vi "macro_LinearSystem_Sim_Execute.vi"() -> ()   [LabVIEW 2019, in "Trajectory_Library.lvlib"]
uses:
  BatterySim_CalculateLoadedBatteryVoltage.vi
  Trajectory_Library.lvlib
  <vilib>/Analysis/Matrix/Datatypes/RealMatrix.ctl
  <vilib>/Analysis/Matrix/NI_Matrix.lvlib
  TypeDef/LINEAR_SYSTEM.ctl
panel:
  in  "Demand Array (CO)":dbl[](array[numeric])
  in  "Linear System":T1
  in  "Current":dbl
  # "<States,States>"
  # "<States,Inputs>"
  # "<Outputs,States>"
  # "<Outputs,Inputs>"
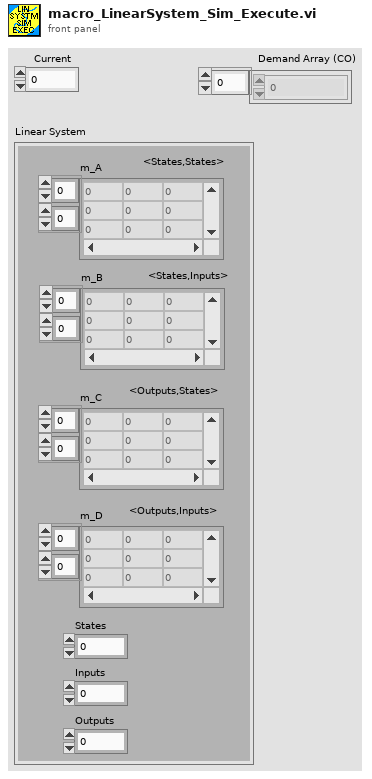
[diagram p1: front panel]
types:
  T1 = typedef "Trajectory_Library.lvlib/LINEAR_SYSTEM.ctl" = cluster{"m_A":T2, "m_B":T2, "m_C":T2, "m_D":T2, "States":i32, "Inputs":i32, "Outputs":i32}
  T2 = typedef "NI_Matrix.lvlib/RealMatrix.ctl" = dbl[][]
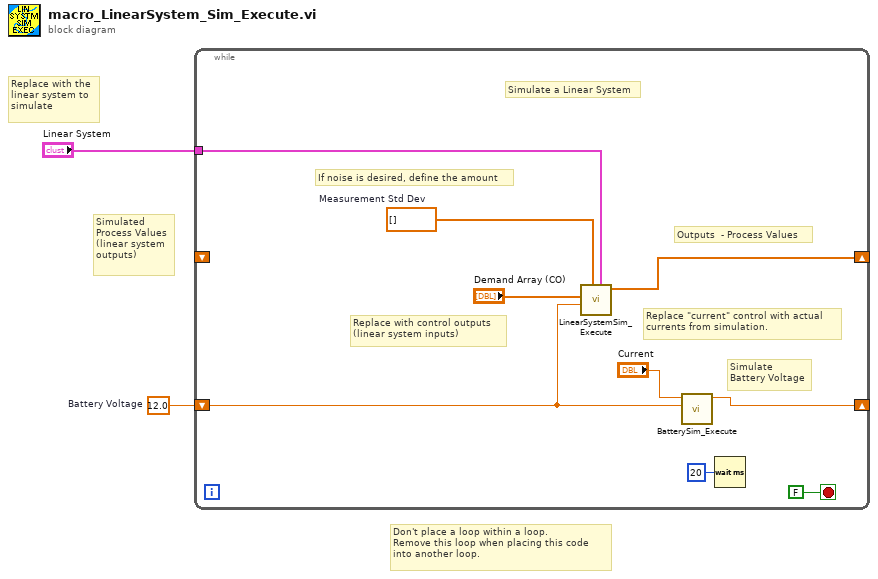
[diagram p0: block diagram]
diagram:
  w2 = 12.0  # Battery Voltage
  # "Replace with the\nlinear system to \nsimulate"
  # "Don't place a loop within a loop. \nRemove this loop when placing this code\ninto another loop."
  # "Simulated\nProcess Values\n(linear system\noutputs)"
  n1 = while {
    shift-right: [w9] -> _
    shift-left: w2 -> [w7]
    shift-right: [w8] -> _
    shift-left: _ -> [_]
    tunnel: "Linear System" -> [w5]
    stop <- FALSE stop-if-true
    w4 = dbl[] []  # Measurement Std Dev
    # "If noise is desired, define the amount"
    # "Replace \"current\" control with actual\ncurrents from simulation."
    # "Outputs  - Process Values"
    # "Replace with control outputs\n(linear system inputs)"
    # "Simulate\nBattery Voltage"
    # "Simulate a Linear System"
    n2 = call "LinearSystemSim_Execute.vi"("Linear System"=w5, "Measurement Std Dev"=w4, "Battery Voltage"=w7, "Demand Array (CO)"="Demand Array (CO)") -> ("Outputs"=w8:dbl[])  [unwired: 5 in, 2 out]
    n3 = call "BatterySim_Execute.vi"("Nominal Battery Voltage"=w7, "Current"="Current") -> ("Voltage"=w9:dbl)  [unwired: 9 in]
    n4 = Wait (ms)(milliseconds to wait=u32 20) -> ()  [unwired: 1 out]
  }
